vi "Get Show_Error_Window.vi"(8 "error in (no error)":errorcluster, 11 "Settings in":refnum<class "Settings.lvclass">) -> (0 "error out":errorcluster, 2 "Show_Error_Window":T1, 3 "Settings out":refnum<class "Settings.lvclass">)   [LabVIEW 2023, in "Error Manager.lvlib" / "Settings.lvclass"]
uses:
  Settings.lvclass
  Settings.lvclass/Settings.ctl
  Show_Error_Window_Setting (enum).ctl
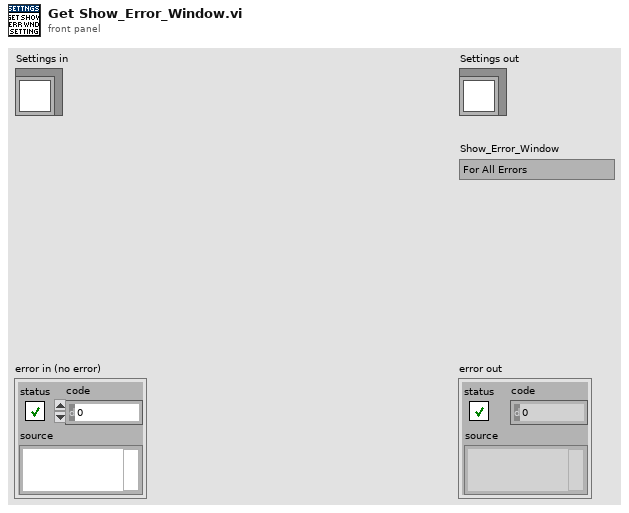
[diagram p1: front panel]
types:
  T1 = typedef "Error Manager.lvlib/Settings.lvclass/Show_Error_Window_Setting (enum).ctl" = enum16{"For All Errors", "For New Errors", "For New Error Codes", "Never"}
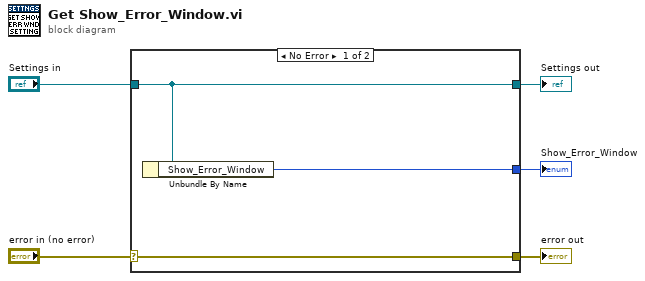
[diagram p0: block diagram]
diagram:
  n1 = case shown="No Error" "error in (no error)" {
    selector: "error in (no error)" -> [w8 w9]
    tunnel: [w8 w9] -> w4
    tunnel: [w7 w10] -> w2
    tunnel: "Settings in" -> [w7 w10]
    tunnel: [w6 _] -> w1
    frame No Error {
      n2 = Unbundle By Name(w7) -> ("Show_Error_Window"=w6:T1)
    }
    frame Error {
    }
  }
  "error out" <- w4
  "Settings out" <- w2
  "Show_Error_Window" <- w1
